vi "ZMC Flash Writef.vi"(7 "pfvlue":sgl, 8 "error in (no error)":errorcluster caption="错误输入（无错误）", 9 "uinumes":u32, 10 "uiflashid":u16, 11 "handle":u32) -> (0 "error out":errorcluster caption="错误输出", 2 "function return":i32, 3 "handle out":u32, 5 "pfvlue out":sgl)   [LabVIEW 2015, in "zauxdll.lvlib"]
doc: "int32 __stdcall ZMC_FlashWritef(ZMC_HANDLE handle, uint16 uiflashid, uint32 uinumes, float *pfvlue);"
uses:
  zauxdll.lvlib
  zmotion.dll
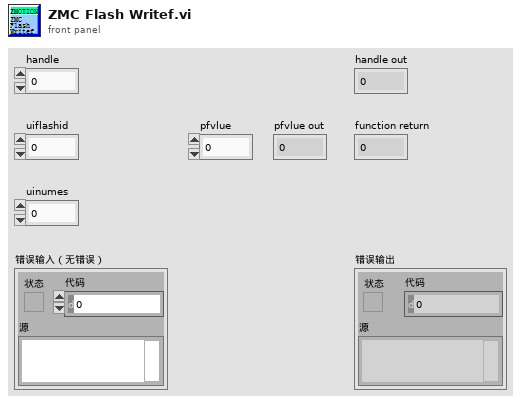
[diagram p1: front panel]
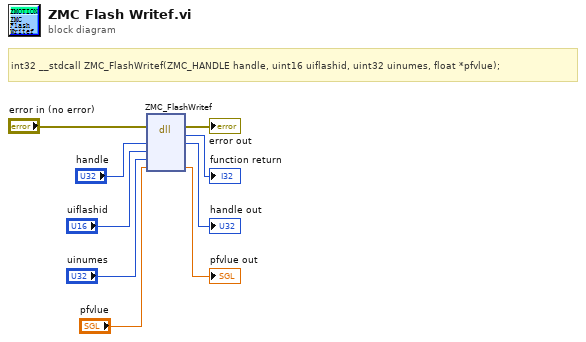
[diagram p0: block diagram]
diagram:
  # "int32 __stdcall ZMC_FlashWritef(ZMC_HANDLE handle, uint16 uiflashid, uint32 uinumes, float *pfvlue);"
  n1 = dll-call lib="C:/Users/VIC/Desktop/GOGORO_SA/system/LLB/zmotion/zaux/zmotion.*" fn="ZMC_FlashWritef"(error in="error in (no error)", "handle"="handle", "uiflashid"="uiflashid", "uinumes"="uinumes", "pfvlue"="pfvlue") -> (error out=→"error out":errorcluster, →"function return":i32, "handle"=→"handle out":u32, "pfvlue"=→"pfvlue out":sgl)  [unwired: 4 in, 1 out]
